vi "Get list of Groups Assigned.vi"(4 "error in (no error)":errorcluster, 7 "VISA resource name":refnum<visa-resource-name>) -> (0 "error out":errorcluster, 2 "List of Groups":string, 3 "VISA resource name out":refnum<visa-resource-name>)   [LabVIEW 2020, in "Newport ESP301.lvlib"]
doc: "This command is used to read the group numbers that have already been created or assigned.\nIf no group have been created returns error"
uses:
  Newport ESP301.lvlib
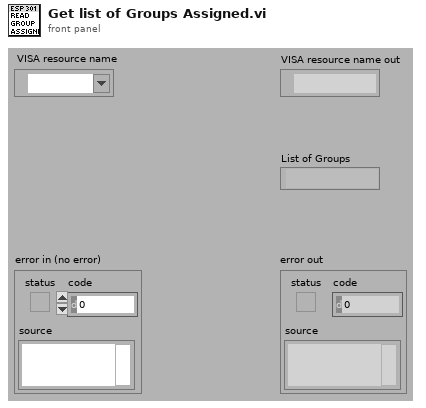
[diagram p1: front panel]
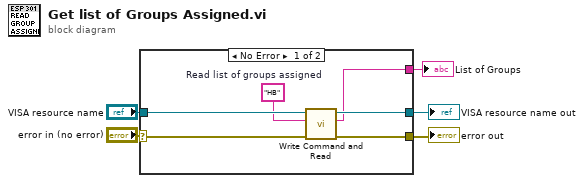
[diagram p0: block diagram]
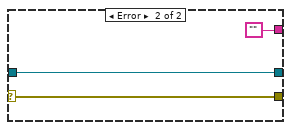
[diagram p2: hidden frame]
diagram:
  n1 = case shown="No Error" "error in (no error)" {
    selector: "error in (no error)" -> [w8 w14]
    tunnel: [w10 w14] -> w5
    tunnel: "VISA resource name" -> [w11 w13]
    tunnel: [w9 w13] -> w4
    tunnel: [w6 ""] -> w1
    frame No Error {
      w7 = "HB"  # Read list of groups assigned
      n2 = call "Write Command and Read.vi"("error in (no error)"=w8, "Command"=w7, "VISA resource name"=w11) -> ("error out"=w10:errorcluster, "Returned string"=w6:string, "VISA resource name out"=w9:refnum<visa-resource-name>)  [unwired: 4 in]
    }
    frame Error {
    }
  }
  "error out" <- w5
  "VISA resource name out" <- w4
  "List of Groups" <- w1
